vi "WriteHeaderAndDataFile.vi"(0 "filename":string, 1 "Array":dbl[][](array[numeric]), 2 "Header":string="1st row: time (ms)\n2nd row: Voltage (V)") -> ()   [LabVIEW 2017]
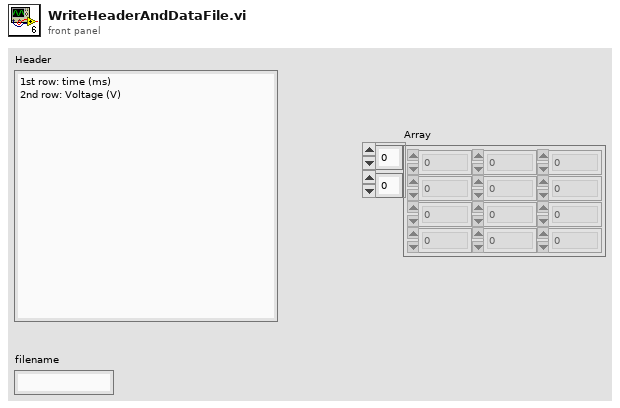
[diagram p1: front panel]
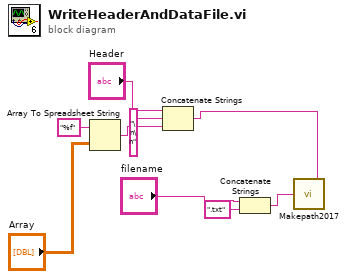
[diagram p0: block diagram]
diagram:
  n1 = Array To Spreadsheet String(array="Array", 3:"%f" ("format string")) -> (spreadsheet string=w8:string)  [unwired: 1 in]
  n2 = Concatenate Strings("Header", "\n\n" ("string"), w8) -> (w7:string)
  n3 = Concatenate Strings("filename", ".txt" ("string")) -> (w3:string)
  n4 = call "Makepath2017.vi"("text to save"=w7, "File name, format \\filename"=w3) -> ()
